vi "pissssssston.vi"(1 "bouton\nbouton":bool) -> ()   [LabVIEW 2018]
uses:
  <vilib>/Rock Robotics/WPI/Solenoid/WPI_SolenoidValue.ctl
  <vilib>/Rock Robotics/WPI/Solenoid/WPI_SolenoidSetEnum.vi
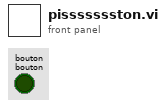
[diagram p1: front panel]
types:
  T1 = typedef "WPI_SolenoidValue.ctl" = enum16{"Off", "On", "Forward", "Reverse"}
  T2 = typedef "WPI_SolenoidDevRef.ctl" = cluster{"DevStatus":errorcluster, "Pneumatics Control Module":u8, "Forward Solenoid Channel":T3, "Reverse Solenoid Channel":T3}
  T3 = typedef "WPI_SolenoidChannel.ctl" = enum8{"Solenoid 0", "Solenoid 1", "Solenoid 2", "Solenoid 3", "Solenoid 4", "Solenoid 5", "Solenoid 6", "Solenoid 7", "Invalid"}
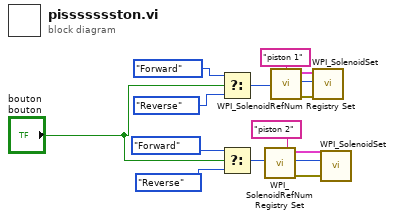
[diagram p0: block diagram]
diagram:
  n1 = Select(t=WPI_SolenoidValue."Forward" ("Value"), s="bouton\nbouton", f=WPI_SolenoidValue."Reverse" ("Value")) -> (s? t:f=w11:T1)
  n2 = Select(t=WPI_SolenoidValue."Forward" ("Value"), s="bouton\nbouton", f=WPI_SolenoidValue."Reverse" ("Value")) -> (s? t:f=w6:T1)
  n3 = call <vilib>:"WPI_SolenoidRefNum Registry Set.vi"("refnum name"="piston 2") -> ("error out"=w3:errorcluster, "SolenoidDevRef"=w4:T2)  [unwired: 9 in]
  n4 = call <vilib>:"WPI_SolenoidRefNum Registry Set.vi"("refnum name"="piston 1") -> ("error out"=w1:errorcluster, "SolenoidDevRef"=w2:T2)  [unwired: 9 in]
  n5 = call-poly <vilib>:"WPI_SolenoidSet.vi"("error in (no error)"=w1, "Value"=w11, "SolenoidDevRef"=w2) -> ()  [unwired: 7 in, 2 out]
  n6 = call-poly <vilib>:"WPI_SolenoidSet.vi"("error in (no error)"=w3, "Value"=w6, "SolenoidDevRef"=w4) -> ()  [unwired: 7 in, 2 out]
